vi "TCP Socket Server.vi"() -> ()   [LabVIEW 2019, in "ANODE Tests.lvlib"]
uses:
  ANODE Tests.lvlib
  Echo Handler/Echo Handler.lvclass
  C:/Users/Nicholas Folse/Documents/workspace/github-tauterra.llc/ANODE/ANODE/Socket API/Connection Handler/Connection Handler.lvclass
  ANODE/Utility API/Log Service/public/level.ctl
  54dd512a-dce5-4669-9818-343de6f004db.vi
  ANODE/Utility API/Queue Log Provider/Queue Log Provider.lvclass
  C:/Users/Nicholas Folse/Documents/workspace/github-tauterra.llc/ANODE/ANODE/Utility API/Log Service/Log Service.lvclass
  ANODE/Socket API/TCP Connection/TCP Connection.lvclass
  ANODE/Socket API/TCP Socket Server/TCP Socket Server.lvclass
  ANODE/Utility API/Log Service/Log Service.lvclass
panel:
  in  "max connections (-1:unlimited)":i32=10
  out "connection count":i32
  out "TCP client error":errorcluster
  out "response time":timestamp
  out "response":string
  in  "send message":bool
  in  "test message":string(combo)="hello"
  out "log":i32(listbox)
  # "Echo Server Test"
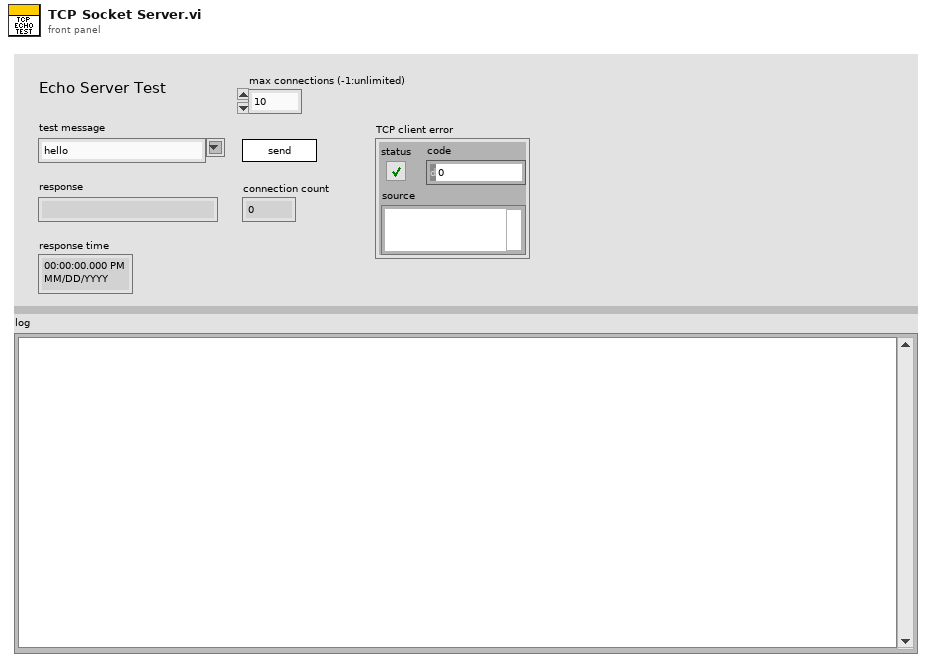
[diagram p1: front panel]
types:
  T1 = typedef "Utility API.lvlib/Log Service.lvclass/level.ctl" = u16
  T2 = enum16{"Standard", "Buffered", "CRLF", "Immediate"}
  T3 = typedef "Queue Log Provider.lvclass/log_message.ctl" = cluster{"Time Stamp":timestamp, "level":T1, "context":string, "message":string}
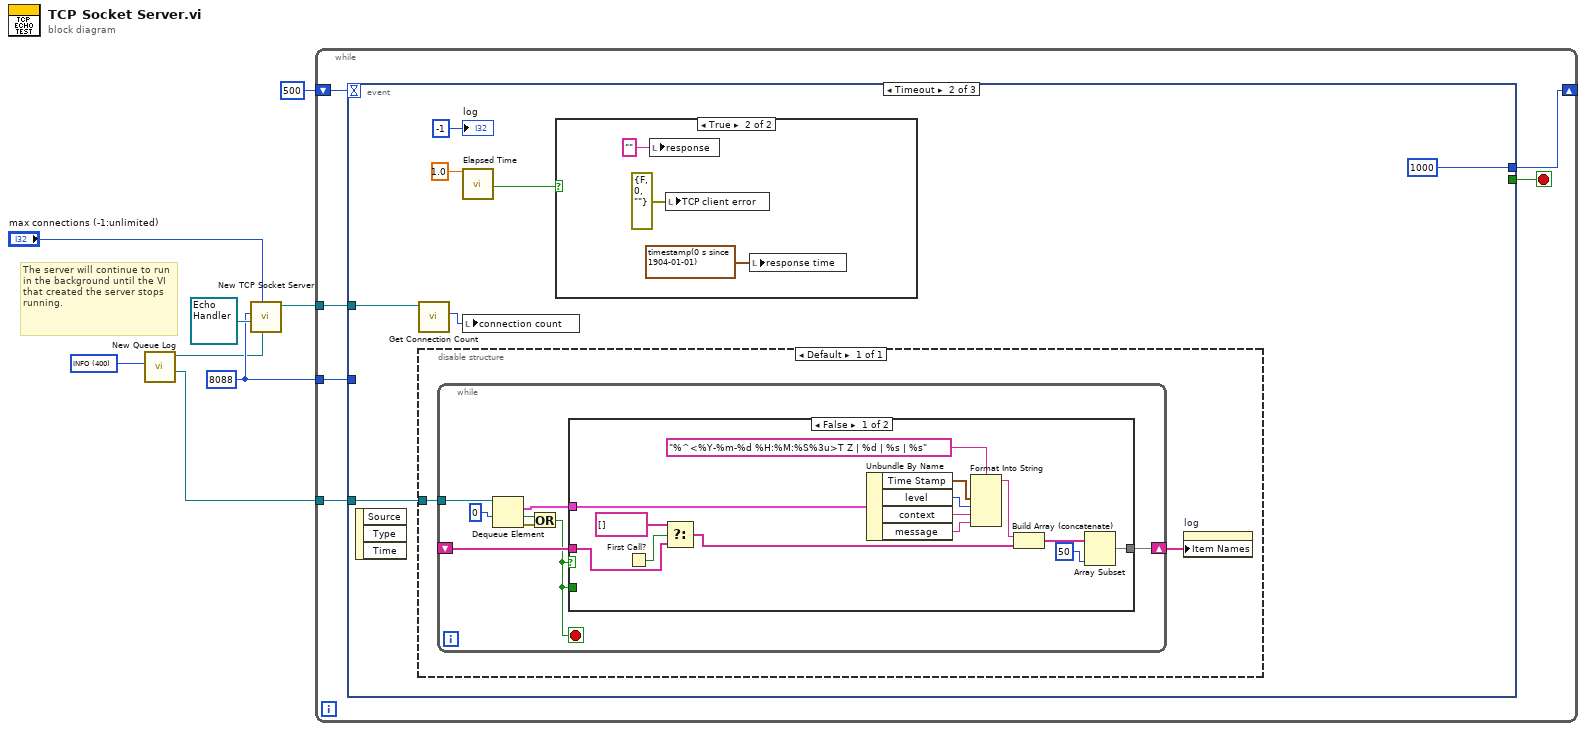
[diagram p0: block diagram]
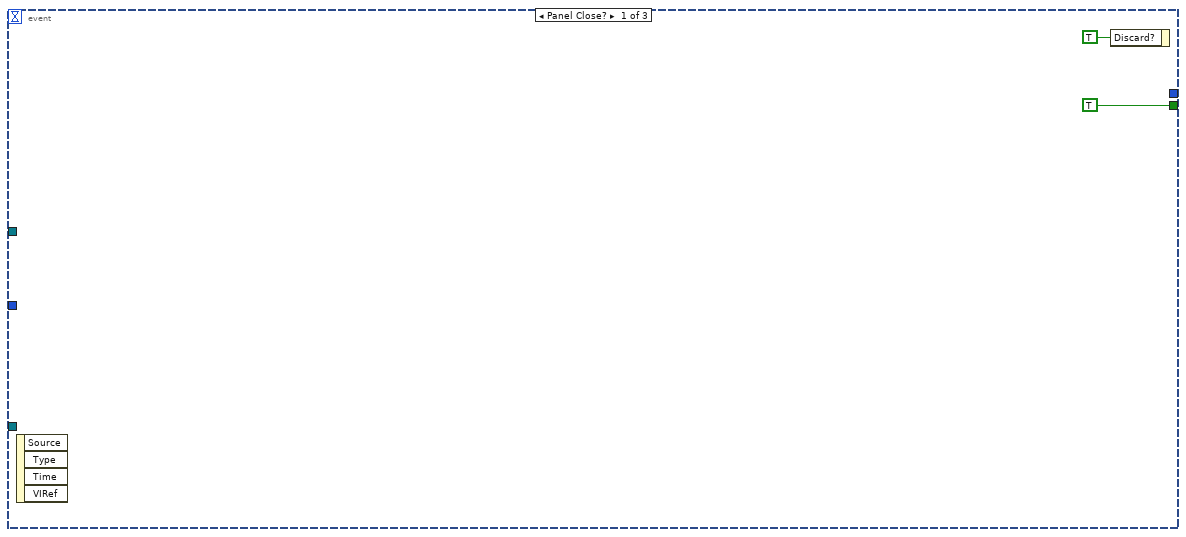
[diagram p2: hidden frame]
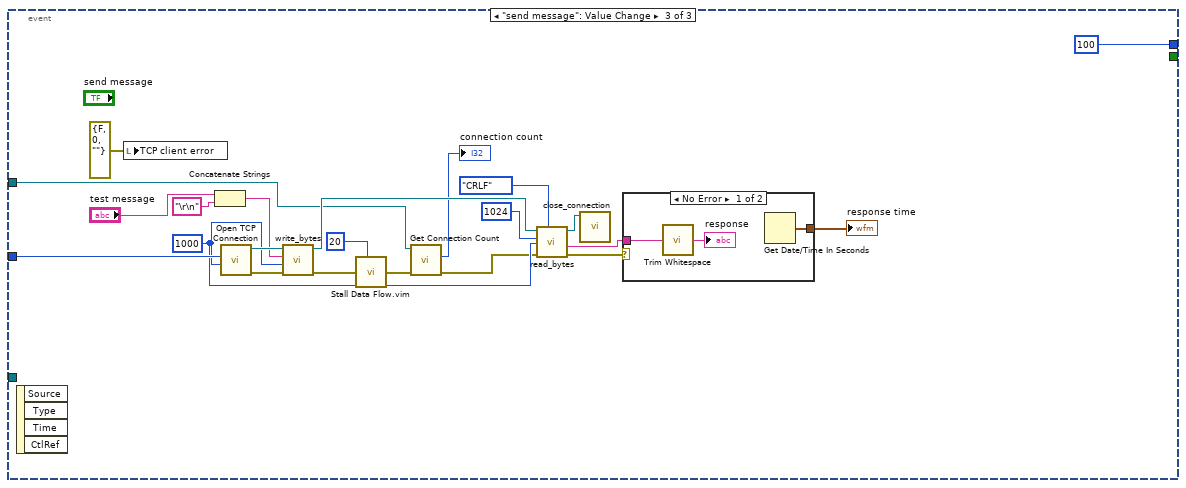
[diagram p5: hidden frame]
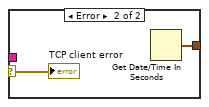
[diagram p6: hidden frame]
diagram:
  w3 = T1 400 items=["OFF"=0, "FATAL"=100, "ERROR"=200, "WARN"=300, "INFO"=400, "DEBUG"=500, "TRACE"=600, "ALL"=65535] ("level")
  w6 = u16 8088 ("port")
  # "The server will continue to run in the background until the VI that created the server stops running."
  n1 = call "New Queue Log.vi"("level"=w3) -> ("queue out"=w4:refnum<queue>, "Queue Log Provider"=w5:refnum<data-value>)  [unwired: 8 in, 1 out]
  n2 = call "New TCP Socket Server.vi"("log service"=w5, "max connections (-1:unlimited)"="max connections (-1:unlimited)", "Connection Handler"=refnum<class "Echo Handler.lvclass"> refnum ("ANODE Tests.lvlib:Echo Handler.lvclass"), "port"=w6) -> ("TCP Server"=w7:refnum<data-value>)  [unwired: 6 in, 1 out]
  n3 = while {
    tunnel: w7 -> [w12]
    tunnel: w6 -> [w13]
    tunnel: w4 -> [w11]
    shift-right: [w10] -> _
    shift-left: 500 -> [w9]
    stop <- w14 stop-if-true
    n4 = event shown="[1] Timeout" {
      selector: _ -> [_ _ _]
      dyn-events: _ -> [_ _ _]
      timeout: w9 -> [_ _ _]
      tunnel: [TRUE ("Discard?") _ _] -> w14
      tunnel: w13 -> [_ _ w69]
      tunnel: w12 -> [_ w23 w59]
      tunnel: w11 -> [_ w19 _]
      tunnel: [_ 1000 100] -> w10
      event Panel Close? {
        n5 = event-data() -> ()  [unwired: 1 in, 4 out]
        n6 = event-data("Discard?"=TRUE) -> ()  [unwired: 1 in, 1 out]
      }
      event Timeout {
        n7 = event-data() -> ()  [unwired: 1 in, 3 out]
        n8 = call "Get Connection Count.vi"("TCP Socket Server in"=w23) -> ("connection count"=w22:i32)  [unwired: 8 in, 2 out]
        n9 = disable-structure shown="Default" {
          disable-tunnel: w19 -> [w25]
          frame Enabled {
            n10 = while {
              tunnel: w25 -> [w33]
              shift-right: [w29] -> w24
              shift-left: _ -> [w28]
              stop <- w26 stop-if-true
              n11 = Dequeue Element(queue=w33, timeout in ms (-1)=0) -> (element=w27:T3, timed out?=w31:bool, error out=w30:errorcluster)  [unwired: 1 in, 1 out]
              n12 = Or(x=w31, y=w30) -> (x .or. y?=w26:bool)
              n13 = case shown="False" w26 {
                tunnel: [w47 w48] -> w29
                tunnel: w26 -> [_ _]
                tunnel: w28 -> [w46 w48]
                tunnel: w27 -> [w45 _]
                frame False {
                  n14 = First Call?() -> (First Call?: T/F=w44:bool)
                  n15 = Select(t=string[] [], s=w44, f=w46) -> (s? t:f=w43:string[])
                  n16 = Unbundle By Name(w45) -> ("Time Stamp"=w40:timestamp, "level"=w39:T1, "context"=w38:string, "message"=w37:string)
                  n17 = Format Into String(format string="%^<%Y-%m-%d %H:%M:%S%3u>T Z | %d | %s | %s", w40, w39, w38, w37) -> (resulting string=w36:string)  [unwired: 2 in, 1 out]
                  n18 = Build Array (concatenate)(w36, w43) -> (w35:string[])
                  n19 = Array Subset(array=w35, length=50) -> (w47:string[])  [unwired: 1 in]
                }
                frame True {
                }
              }
            }
            n20 = property on="log" class="LstBox (strict)"("Item Names"=w24) -> ()  [unwired: 2 in, 2 out]
          }
        }
        n21 = call "Elapsed Time"("Time Target (s)"=1.0) -> ("Time has Elapsed"=w20:bool)  [unwired: 11 in, 7 out]
        n22 = local write "connection count"(w22) -> ()
        n23 = case shown="True" w20 {
          frame False {
          }
          frame True {
            n24 = local write "response"("" ("response")) -> ()
            n25 = local write "TCP client error"(errorcluster {"status"=FALSE, "code"=0, "source"=""} ("TCP client error")) -> ()
            n26 = local write "response time"(timestamp(0 s since 1904-01-01)) -> ()
          }
        }
        "log" <- -1 ("log")
      }
      event "send message": Value Change {
        w63 = 1000 ("timeout ms (60000)")
        n27 = event-data() -> ()  [unwired: 1 in, 4 out]
        n28 = local write "TCP client error"(errorcluster {"status"=FALSE, "code"=0, "source"=""} ("TCP client error")) -> ()
        n29 = Concatenate Strings("test message", "\r\n" ("string")) -> (w65:string)
        n30 = call "Open TCP Connection.vi"("timeout ms (60000)"=w63, "remote port"=w69) -> ("error out"=w66:errorcluster, "TCP Connection out"=w67:refnum<class "TCP Connection.lvclass">)  [unwired: 8 in]
        n31 = call-dynamic "write_bytes.vi"("error in (no error)"=w66, "timeout ms (-1)"=w63, "data in"=w65, "TCP Connection in"=w67) -> ("error out"=w55:errorcluster, "TCP Connection out"=w64:refnum<class "TCP Connection.lvclass">)  [unwired: 4 in, 2 out]
        n32 = call "Stall Data Flow.vim"("value in"=w55, "milliseconds to wait"=u32 20) -> ("value out"=w54:errorcluster)  [unwired: 1 out]
        n33 = call "Get Connection Count.vi"("error in (no error)"=w54, "TCP Socket Server in"=w59) -> ("error out"=w58:errorcluster, "connection count"=→"connection count":i32)  [unwired: 7 in, 1 out]
        n34 = call-dynamic "read_bytes.vi"("read mode"=T2."CRLF" ("mode (standard)"), "error in (no error)"=w58, "timeout (ms)"=w63, "bytes to read"=1024, "TCP Connection in"=w64) -> ("error out"=w62:errorcluster, "data out"=w61:string, "TCP Connection out"=w56:refnum<class "TCP Connection.lvclass">)  [unwired: 3 in, 1 out]
        n35 = call-dynamic "close_connection.vi"("TCP Connection in"=w56) -> ()  [unwired: 10 in, 1 out]
        n36 = case shown="No Error" w62 {
          selector: w62 -> [_ w78]
          tunnel: w61 -> [w76 _]
          tunnel: [w75 w77] -> w70
          frame No Error {
            n37 = call <vilib>:"Trim Whitespace.vi"("string"=w76) -> ("trimmed string"=→"response":string)  [unwired: 1 in]
            n38 = Get Date/Time In Seconds() -> (seconds since 1Jan1904=w75:timestamp)
          }
          frame Error {
            n39 = Get Date/Time In Seconds() -> (seconds since 1Jan1904=w77:timestamp)
            "TCP client error" <- w78
          }
        }
        "response time" <- w70
      }
    }
  }
